vi "hmi_start_enable.vi"(7 "hmi_references":T1, 8 "error in (no error)":errorcluster) -> (0 "error out":errorcluster)   [LabVIEW 2015, in "lv-build-interface.lvlib"]
uses:
  lv-build-interface.lvlib
  _controls/hmi_references.ctl
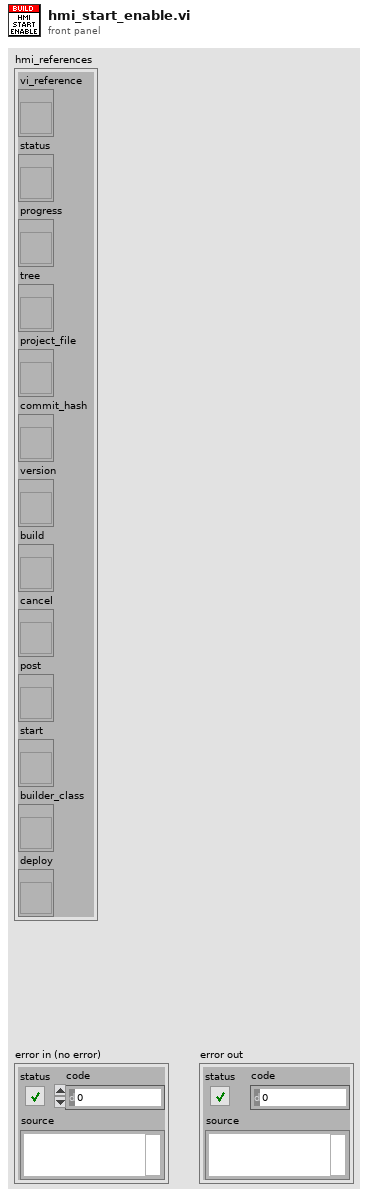
[diagram p1: front panel]
types:
  T1 = typedef "lv-build-interface.lvlib/hmi_references.ctl" = cluster{"vi_reference":refnum<vi>, "status":refnum<vi>, "progress":refnum<vi>, "tree":refnum<vi>, "project_file":refnum<vi>, "commit_hash":refnum<vi>, "version":refnum<vi>, "build":refnum<vi>, "cancel":refnum<vi>, "post":refnum<vi>, "start":refnum<vi>, "builder_class":refnum<vi>, "deploy":refnum<vi>}
  T2 = enum8{"Enabled", "Disabled", "Disabled and Grayed Out"}
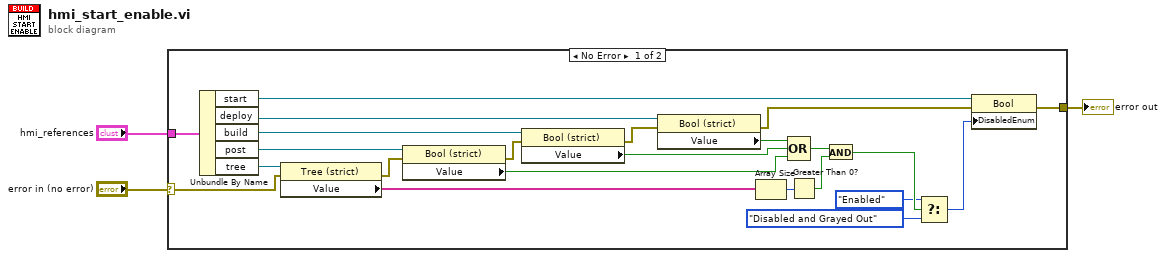
[diagram p0: block diagram]
diagram:
  n1 = case shown="No Error" "error in (no error)" {
    selector: "error in (no error)" -> [w25 w27]
    tunnel: "hmi_references" -> [w22 _]
    tunnel: [w18 w27] -> w1
    frame No Error {
      n2 = Unbundle By Name(w22) -> ("start"=w26:refnum<vi>, "deploy"=w7:refnum<vi>, "build"=w13:refnum<vi>, "post"=w12:refnum<vi>, "tree"=w23:refnum<vi>)
      n3 = property class="Tree (strict)"(reference=w23, error in=w25) -> (error out=w10:errorcluster, "Value"=w24:string[])  [unwired: 1 out]
      n4 = property class="Bool (strict)"(reference=w12, error in=w10) -> (error out=w11:errorcluster, "Value"=w9:bool)  [unwired: 1 out]
      n5 = property class="Bool (strict)"(reference=w13, error in=w11) -> (error out=w6:errorcluster, "Value"=w8:bool)  [unwired: 1 out]
      n6 = property class="Bool (strict)"(reference=w7, error in=w6) -> (error out=w5:errorcluster, "Value"=w4:bool)  [unwired: 1 out]
      n7 = Array Size(array=w24) -> (size(s)=w20:i32)
      n8 = Compound Arithmetic op=OR(w4, w8, w9) -> (w14:bool)
      n9 = Greater Than 0?(x=w20) -> (x > 0?=w21:bool)
      n10 = And(x=w14, y=w21) -> (x .and. y?=w19:bool)
      n11 = Select(t=T2."Enabled" ("Disabled"), s=w19, f=T2."Disabled and Grayed Out" ("Disabled")) -> (s? t:f=w17:T2)
      n12 = property on="Property Node" class="Bool"(reference=w26, error in=w5, "DisabledEnum"=w17) -> (error out=w18:errorcluster)  [unwired: 1 out]
    }
    frame Error {
    }
  }
  "error out" <- w1
